vi "2D_scan.vi"(0 "Y DELAY (ms)":u32=30, 1 "Y Samples":u16=100 min=1 step=1, 2 "Y End  (um)":dbl=100.0 min=0.0 max=100.0 step=0.2 format="%.3f", 3 "Y Start  (um)":dbl min=0.0 max=100.0 step=0.5 format="%.3f", 7 "Outgoing Handle":i32, 8 "X DELAY (ms)":u32=10, 9 "X Samples":u16=100 min=1 step=1, 10 "X End  (um)":dbl=100.0 min=0.0 max=100.0 step=0.2 format="%.3f", 11 "X Start  (um)":dbl min=0.0 max=100.0 step=0.5 format="%.3f") -> ()   [LabVIEW 2013]
uses:
  <instrlib>/Mad_City_2D/MADLib.dll
panel:
  out "X Position (um)":dbl(graph)
  out "Y Position (um)":dbl(graph)
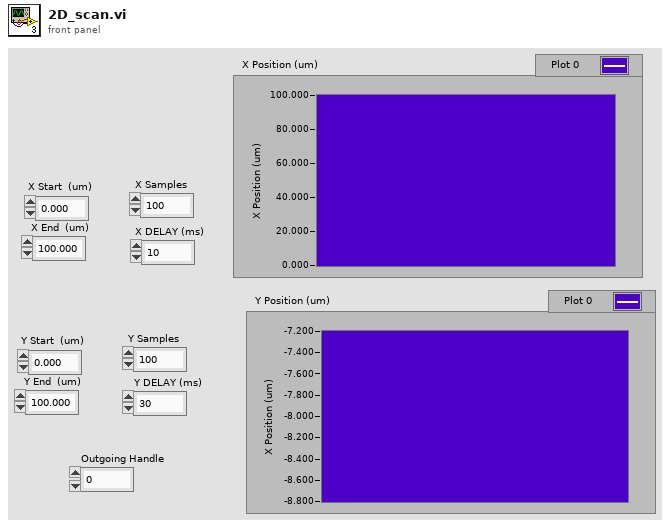
[diagram p1: front panel]
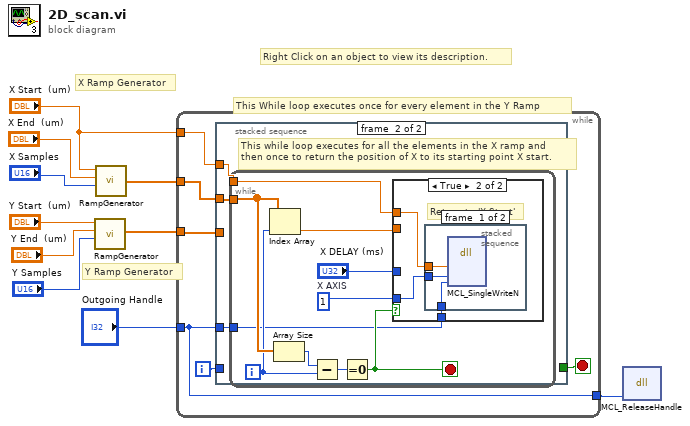
[diagram p0: block diagram]
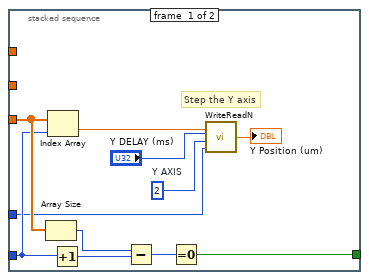
[diagram p2: hidden frame]
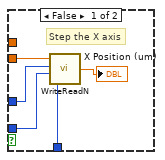
[diagram p3: hidden frame]
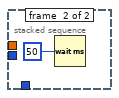
[diagram p4: hidden frame]
diagram:
  # "This While loop executes once for every element in the Y Ramp"
  # "Right Click on an object to view its description."
  # "X Ramp Generator"
  # "Y Ramp Generator"
  n1 = call <instrlib>:"RampGenerator.vi"("Number of Positions"="Y Samples", "End  (um)"="Y End  (um)", "Start  (um)"="Y Start  (um)") -> ("Array"=w4:dbl[])  [unwired: 1 in]
  n2 = call <instrlib>:"RampGenerator.vi"("Number of Positions"="X Samples", "End  (um)"="X End  (um)", "Start  (um)"="X Start  (um)") -> ("Array"=w10:dbl[])  [unwired: 1 in]
  n3 = while {
    tunnel: w10 -> [w15]
    tunnel: w4 -> [w16]
    tunnel: "X Start  (um)" -> [w12]
    tunnel: "Outgoing Handle" -> [w11]
    tunnel: [w11] -> w2
    i -> [w13]
    stop <- w14 stop-if-true
    # "X Ramp Generator"
    n4 = stacked-sequence {
      tunnel: w16 -> [w27 _]
      tunnel: [w25 _] -> w14
      tunnel: w13 -> [w21 _]
      tunnel: w15 -> [_ w30]
      tunnel: w12 -> [_ w29]
      tunnel: w11 -> [w17 w28]
      frame #0 {
        w22 = 2  # Y AXIS
        # "Step the Y axis"
        n5 = Array Size(array=w27) -> (size(s)=w24:i32)
        n6 = Index Array(array=w27, index=w21) -> (element=w18:dbl)
        n7 = Increment(x=w21) -> (x+1=w20:i32)
        n8 = Subtract(x=w24, y=w20) -> (x-y=w26:i32)
        n9 = Equal To 0?(x=w26) -> (x = 0?=w25:bool)
        n10 = call <instrlib>:"WriteReadN.vi"("Handle"=w17, "Axis"=w22, "Delay (ms)"="Y DELAY (ms)", "Move to (um)"=w18) -> ("Current Position (um)"=→"Y Position (um)":dbl)
      }
      frame #1 {
        # "This while loop executes for all the elements in the X ramp and \nthen once to return the position of X to its starting point X start."
        n11 = while {
          tunnel: w30 -> [w38]
          tunnel: w29 -> [w33]
          tunnel: w28 -> [w31]
          i -> [w36]
          stop <- w37 stop-if-true
          w34 = 1  # X AXIS
          n12 = Index Array(array=w38, index=w36) -> (element=w32:dbl)
          n13 = Array Size(array=w38) -> (size(s)=w39:i32)
          n14 = Subtract(x=w39, y=w36) -> (x-y=w40:i32)
          n15 = Equal To 0?(x=w40) -> (x = 0?=w37:bool)
          n16 = case shown="True" w37 {
            tunnel: w32 -> [w44 _]
            tunnel: "X DELAY (ms)" -> [w41 _]
            tunnel: w34 -> [w42 w48]
            tunnel: w33 -> [_ w47]
            tunnel: w31 -> [w43 w46]
            frame False {
              # "Step the X axis"
              n17 = call <instrlib>:"WriteReadN.vi"("Handle"=w43, "Axis"=w42, "Delay (ms)"=w41, "Move to (um)"=w44) -> ("Current Position (um)"=→"X Position (um)":dbl)
            }
            frame True {
              # "Return to 'X Start'"
              # "X AXIS SCAN"
              n18 = stacked-sequence {
                tunnel: w48 -> [w51 _]
                tunnel: w47 -> [w50 _]
                tunnel: w46 -> [w49 _]
                frame #0 {
                  n19 = dll-call lib="C:/Program Files/National Instruments/LabVIEW 2013/instr.lib/Mad_City_2D/MADLib.dll" fn="MCL_SingleWriteN"("position"=w50, "axis"=w51, "handle"=w49) -> ()  [unwired: 7 in, 2 out]
                }
                frame #1 {
                  n20 = Wait (ms)(milliseconds to wait=50) -> ()  [unwired: 1 out]
                }
              }
            }
          }
        }
      }
    }
  }
  n21 = dll-call lib="C:/Program Files/National Instruments/LabVIEW 2013/instr.lib/Mad_City_2D/MADLib.dll" fn="MCL_ReleaseHandle"("handle"=w2) -> ()  [unwired: 5 in, 2 out]
